vi "Ini step result.vi"(9 "index (row)":u32, 10 "new element/subarray":string[](array[string]), 11 "Out Data":string[][](array[string])) -> (3 "output array":string[][](array[string]))   [LabVIEW 2020]
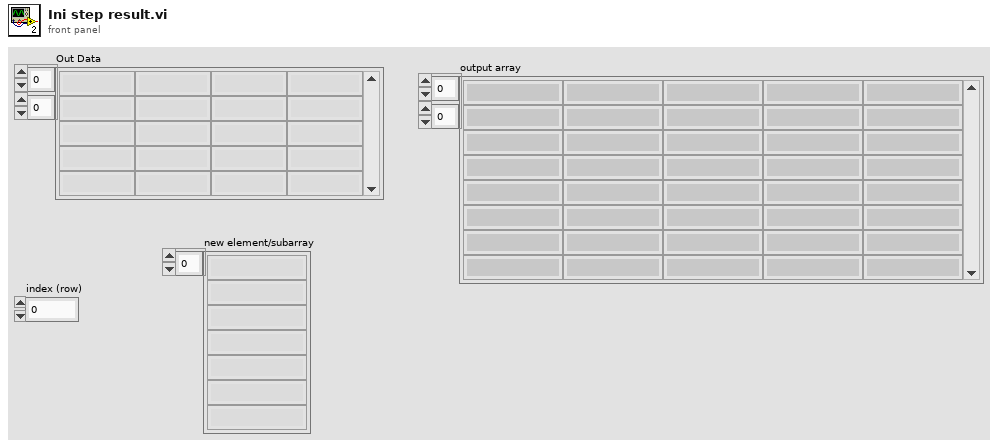
[diagram p1: front panel]
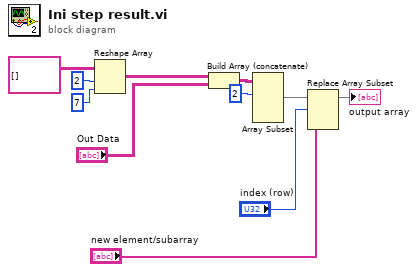
[diagram p0: block diagram]
diagram:
  n1 = Reshape Array(string[][] [] ("array"), 2 ("dimension size"), 7 ("dimension size")) -> (w6:string[][])
  n2 = Build Array (concatenate)(w6, "Out Data") -> (w8:string[][])
  n3 = Array Subset(array=w8, index (row)=2 ("index")) -> (w10:string[][])  [unwired: 3 in]
  n4 = Replace Array Subset(array=w10, new element="new element/subarray", index (row)="index (row)") -> (→"output array":string[][])  [unwired: 1 in]
